vi "GenerateAPIs.vi"() -> ()   [LabVIEW 2017, in "Message Queue.lvlib"]
uses:
  Message Queue.lvlib
  <vilib>/Utility/traverseref.llb/TRef TravTarget.ctl
  <vilib>/Utility/traverseref.llb/VI Scripting - Traverse.lvlib
panel:
  in  "Queue Name":string="UI"
  in  "vi path":path=path "C:/Users/bartl/Downloads/FBIC_3 20190920/FBIC_3 20190920/UI.vi"
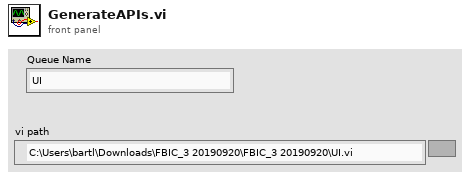
[diagram p1: front panel]
types:
  T1 = typedef "TRef TravTarget.ctl" = enum16{"FP", "BD", "Other"}
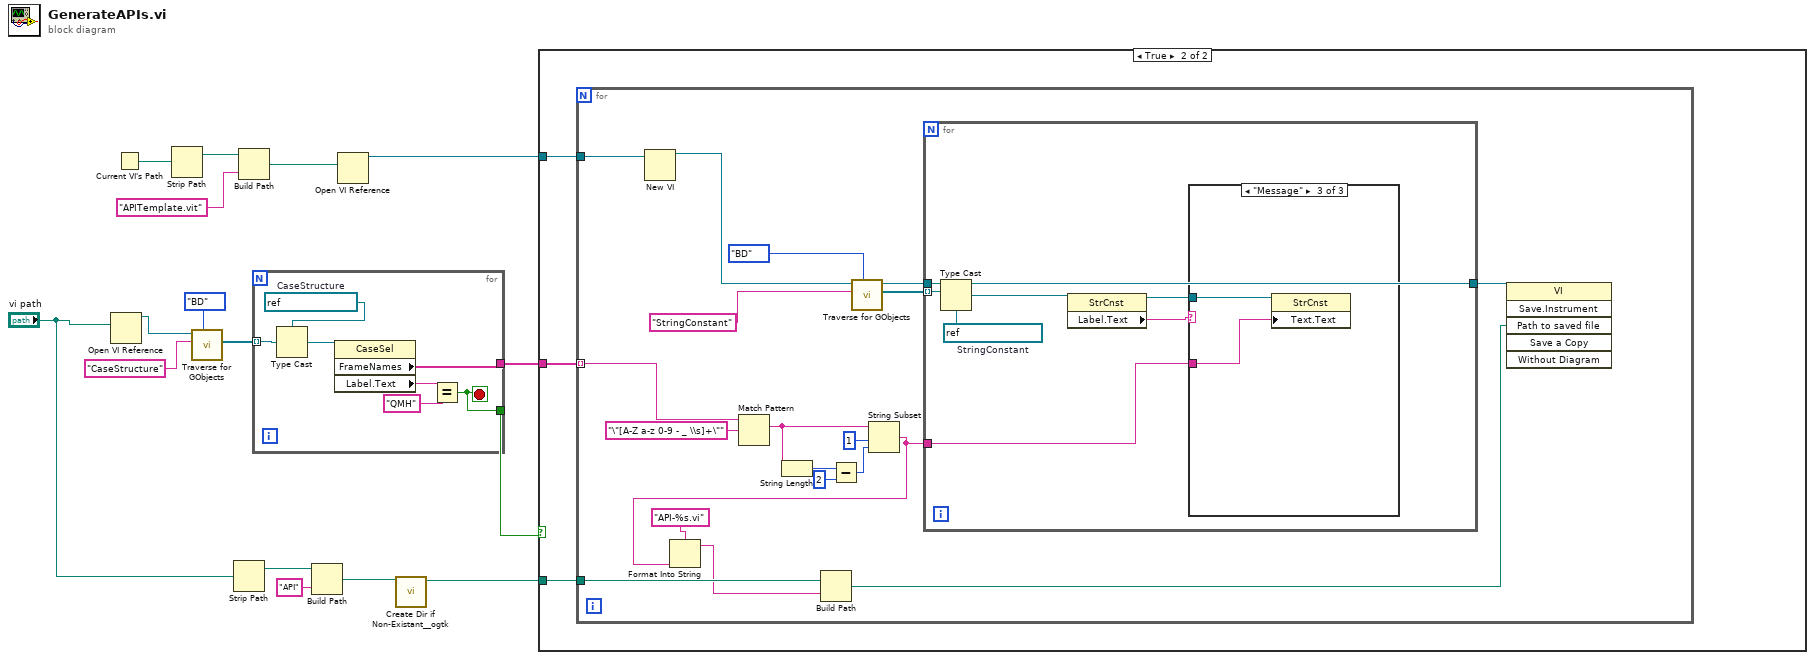
[diagram p0: block diagram]
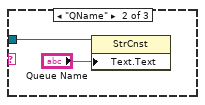
[diagram p4: hidden frame]
diagram:
  n1 = Open VI Reference(vi path="vi path") -> (vi reference=w16:refnum<vi>)  [unwired: 5 in, 1 out]
  n2 = Current VI's Path() -> (path=w12:path)
  n3 = Strip Path(path=w12) -> (stripped path=w11:path)  [unwired: 1 out]
  n4 = call <vilib>:"Traverse for GObjects.vi"("Traverse Target"=TRef_TravTarget."BD", "Class Name"="CaseStructure", "VI Refnum"=w16) -> ("References"=w13:refnum<vi>[])  [unwired: 5 in, 3 out]
  n5 = Strip Path(path="vi path") -> (stripped path=w4:path)  [unwired: 1 out]
  n6 = Build Path(base path=w11, name or relative path="APITemplate.vit") -> (appended path=w9:path)
  n7 = for {
    tunnel: w13 -> [w23] mode=indexing
    tunnel: [w18] -> w7
    tunnel: [w17] -> w8
    stop <- w17 stop-if-true
    w22 = refnum<vi> refnum  # CaseStructure
    n8 = Type Cast(type=w22, x=w23) -> (*(type *) &x=w21:refnum<vi>)
    n9 = property class="CaseSel"(reference=w21) -> ("FrameNames"=w18:string[], "Label.Text"=w20:string)  [unwired: 1 in, 2 out]
    n10 = Equal?(x=w20, y="QMH") -> (x = y?=w17:bool)
  }
  n11 = Build Path(base path=w4, name or relative path="API") -> (appended path=w2:path)
  n12 = Open VI Reference(vi path=w9) -> (vi reference=w6:refnum<vi>)  [unwired: 5 in, 1 out]
  n13 = call <userlib>:"Create Dir if Non-Existant__ogtk.vi"("Directory Path"=w2) -> ("dup Directory Path"=w1:path)  [unwired: 8 in, 2 out]
  n14 = case shown="True" w8 {
    tunnel: w7 -> [_ w26]
    tunnel: w6 -> [_ w25]
    tunnel: w1 -> [_ w24]
    frame False {
    }
    frame True {
      n15 = for {
        tunnel: w26 -> [w28] mode=indexing
        tunnel: w25 -> [w45]
        tunnel: w24 -> [w39]
        n16 = New VI(10:w45) -> (3:w44:refnum<vi>)  [unwired: 6 in, 1 out]
        n17 = Match Pattern(string=w28, regular expression="\"[A-Z a-z 0-9 - _ \\s]+\"") -> (match substring=w32:string)  [unwired: 1 in, 3 out]
        n18 = String Length(string=w32) -> (length=w33:i32)
        n19 = Subtract(x=w33, y=2) -> (x-y=w34:i32)
        n20 = call <vilib>:"Traverse for GObjects.vi"("Traverse Target"=TRef_TravTarget."BD", "Class Name"="StringConstant", "VI Refnum"=w44) -> ("References"=w42:refnum<vi>[], "dup VI Refnum"=w41:refnum<vi>)  [unwired: 5 in, 2 out]
        n21 = String Subset(string=w32, offset (0)=1, length (rest)=w34) -> (substring=w27:string)
        n22 = Format Into String(format string="API-%s.vi", w27) -> (resulting string=w37:string)  [unwired: 2 in, 1 out]
        n23 = Build Path(base path=w39, name or relative path=w37) -> (appended path=w36:path)
        n24 = for {
          tunnel: w42 -> [w52] mode=indexing
          tunnel: w41 -> [w47]
          tunnel: [w47] -> w40
          tunnel: w27 -> [w46]
          w51 = refnum<vi> refnum  # StringConstant
          n25 = Type Cast(type=w51, x=w52) -> (*(type *) &x=w50:refnum<vi>)
          n26 = property class="StrCnst"(reference=w50) -> (reference out=w48:refnum<vi>, "Label.Text"=w49:string)  [unwired: 1 in, 1 out]
          n27 = case shown="\"Message\"" w49 {
            tunnel: w48 -> [_ w54 w56]
            tunnel: w46 -> [_ _ w55]
            frame "False", Default {
            }
            frame "QName" {
              n28 = property class="StrCnst"(reference=w54, "Text.Text"="Queue Name") -> ()  [unwired: 1 in, 2 out]
            }
            frame "Message" {
              n29 = property class="StrCnst"(reference=w56, "Text.Text"=w55) -> ()  [unwired: 1 in, 2 out]
            }
          }
        }
        n30 = invoke class="VI" method="Save.Instrument"(reference=w40, "Path to saved file"=w36) -> ()  [unwired: 4 in, 6 out]
      }
    }
  }
